vi "GetLocalizedPhraseLowLevel.vi"(7 "Dictionary":T1, 8 "error in (no error)":errorcluster, 10 "Target Language":string, 11 "Key":string) -> (0 "error out":errorcluster, 3 "Localized Phrase":string)   [LabVIEW 2017, in "JKI Simple Localization.lvlib"]
uses:
  API/JKI Simple Localization.lvlib
  Definitions/Dictionary--Cluster.ctl
  Definitions/Private/Font -- Cluster.ctl
  Definitions/Private/Phrase Dictionary Entry -- Cluster.ctl
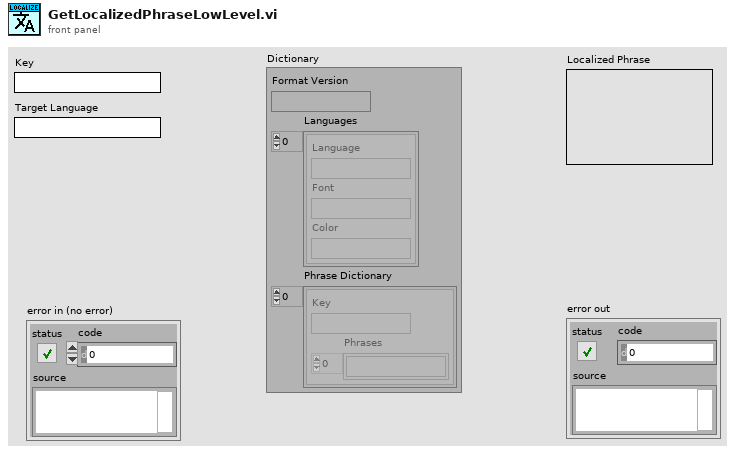
[diagram p1: front panel]
types:
  T1 = typedef "JKI Simple Localization.lvlib/Dictionary--Cluster.ctl" = cluster{"Format Version":string, "Languages":T2[], "Phrase Dictionary":T3[]}
  T2 = typedef "JKI Simple Localization.lvlib/Font -- Cluster.ctl" = cluster{"Language":string, "Font":string, "Color":string}
  T3 = typedef "JKI Simple Localization.lvlib/Phrase Dictionary Entry -- Cluster.ctl" = cluster{"Key":string, "Phrases":string[]}
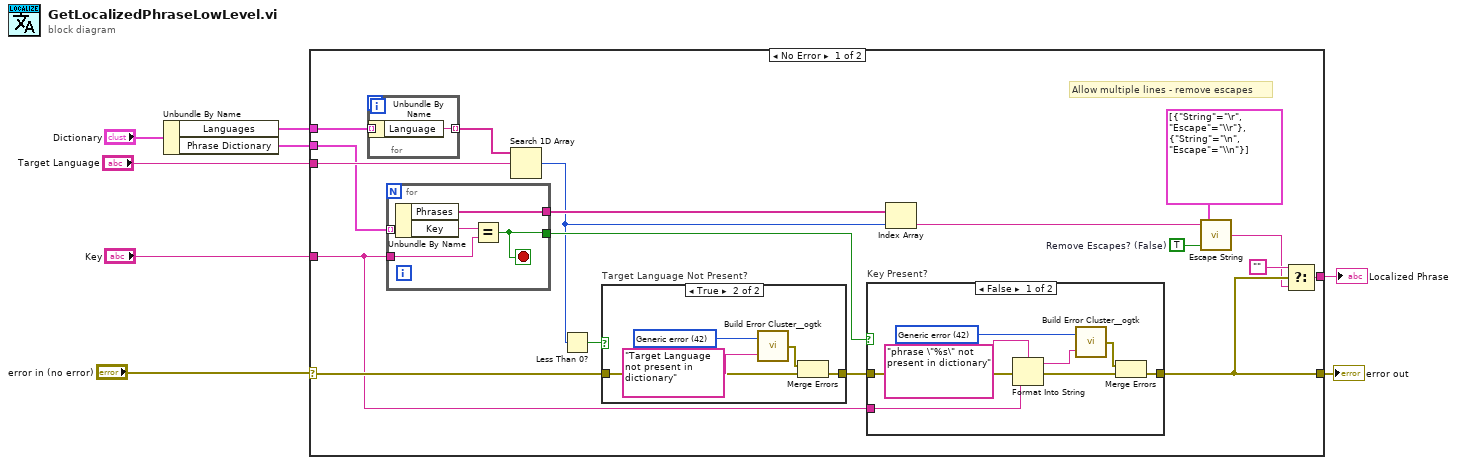
[diagram p0: block diagram]
diagram:
  n1 = Unbundle By Name("Dictionary") -> ("Languages"=w3:T2[], "Phrase Dictionary"=w1:T3[])
  n2 = case shown="No Error" "error in (no error)" {
    selector: "error in (no error)" -> [w22 w49]
    tunnel: w3 -> [w10 _]
    tunnel: [w12 _] -> w8
    tunnel: [w15 w49] -> w7
    tunnel: "Target Language" -> [w21 _]
    tunnel: "Key" -> [w11 _]
    tunnel: w1 -> [w16 _]
    frame No Error {
      w24 = TRUE  # Remove Escapes? (False)
      # "Allow multiple lines - remove escapes"
      n3 = for {
        tunnel: w10 -> [w28] mode=indexing
        tunnel: [w27] -> w9 mode=indexing
        n4 = Unbundle By Name(w28) -> ("Language"=w27:string)
      }
      n5 = for {
        tunnel: w16 -> [w33] mode=indexing
        tunnel: w11 -> [w31]
        tunnel: [w30] -> w19
        tunnel: [w29] -> w20
        stop <- w30 stop-if-true
        n6 = Unbundle By Name(w33) -> ("Phrases"=w29:string[], "Key"=w32:string)
        n7 = Equal?(x=w32, y=w31) -> (x = y?=w30:bool)
      }
      n8 = Search 1D Array(1D array=w9, element=w21) -> (index of element=w18:i32)  [unwired: 1 in]
      n9 = Less Than 0?(x=w18) -> (x < 0?=w26:bool)
      n10 = case "Target Language Not Present?" shown="True" w26 {
        tunnel: w22 -> [w43 w45]
        tunnel: [w43 w44] -> w25
        frame False {
        }
        frame True {
          w48 = 42 items=["No error", "Argument error", "Memory is full", "Out of zone", "End of file", "File already open", "Generic file I/O error", "File not found", "File permission error", "Disk is full", "Duplicate path", "Too many files open", "System feature not enabled", "Resource file not found", "Cannot add resource", "Resource not found", "Image not found", "Image memory error", "Pen does not exist", "Config type invalid", "Config token not found", "Config parse error", "Config memory error", "Bad external code format", "Bad external code offset", "External code not present", "Null window", "Destroy window error", "Null menu", "Print aborted", "Bad print record", "Print driver error", "Windows error during printing", "Memory error during printing", "Print dialog error", "Generic print error", "Invalid device refnum", "Device not found", "Device parameter error", "Device unit error", "Cannot open device", "Device call aborted", "Generic error", "Cancelled by user", "Object ID too low", "Object ID too high", "Object not in heap", "Unknown heap", "Unknown object (invalid DefProc)", "Unknown object (DefProc not in table)", "Message out of range", "Invalid (null) method", "Unknown message", "Manager call not supported", "Bad address", "Network operation in progress", "Network operation timed out", "Connection is busy", "Network attribute not supported", "Network error", "Address in use", "System out of memory", "Connection aborted", "Connection refused", "Not connected", "Already connected", "Connection closed", "Initialization error (interapplication manager)", "Bad occurrence", "Wait on unbound occurrence handler", "Occurrence queue overflow", "Datalog type conflict", "Unused", "Unrecognized type (interapplication manager)", "Memory corrupt", "Failed to make temporary DLL", "Old CIN version", "Drag socket not found", "Failed to load drop-object", "Failed to register OLE object", "Failed to release OLE object", "Format specifier type mismatch", "Unknown format specifier", "Too few format specifiers", "Too many format specifiers", "Scan failed", "Newer CIN version", "Error converting to variant", "Runtime menu error", "Password tampered", "Variant attribute not found", "Incompatible variant data type", "Event data is not available", "Event Store is not present", "Occurrence is not found", "Event Queue is not created", "Event info is not available", "Refnum passed is NULL", "Error retrieving Class GUID", "Error retrieving CoClass GUID", "Error retrieving TypeLib GUID.", "Bad built application magic bytes.", "Specific driver is different from the specific driver associated with the Logical Name.", "There is no session opened to the class driver.", "Max Error", "MAX - Error with config objects", "MAX - Error loading configuration", "MAX - Group not supported"]
          n11 = call <userlib>:"Build Error Cluster__ogtk.vi"("String to Prepend to source (\"\")"="Target Language not present in dictionary" ("String to Prepend to source (\"\")"), "code"=w48) -> ("error out"=w46:errorcluster)
          n12 = Merge Errors(w46, w45) -> (w44:errorcluster)
        }
      }
      n13 = case "Key Present?" shown="False" w19 {
        tunnel: w25 -> [w38 w42]
        tunnel: [w39 w42] -> w15
        tunnel: w11 -> [w35 _]
        frame False {
          w41 = 42 items=["No error", "Argument error", "Memory is full", "Out of zone", "End of file", "File already open", "Generic file I/O error", "File not found", "File permission error", "Disk is full", "Duplicate path", "Too many files open", "System feature not enabled", "Resource file not found", "Cannot add resource", "Resource not found", "Image not found", "Image memory error", "Pen does not exist", "Config type invalid", "Config token not found", "Config parse error", "Config memory error", "Bad external code format", "Bad external code offset", "External code not present", "Null window", "Destroy window error", "Null menu", "Print aborted", "Bad print record", "Print driver error", "Windows error during printing", "Memory error during printing", "Print dialog error", "Generic print error", "Invalid device refnum", "Device not found", "Device parameter error", "Device unit error", "Cannot open device", "Device call aborted", "Generic error", "Cancelled by user", "Object ID too low", "Object ID too high", "Object not in heap", "Unknown heap", "Unknown object (invalid DefProc)", "Unknown object (DefProc not in table)", "Message out of range", "Invalid (null) method", "Unknown message", "Manager call not supported", "Bad address", "Network operation in progress", "Network operation timed out", "Connection is busy", "Network attribute not supported", "Network error", "Address in use", "System out of memory", "Connection aborted", "Connection refused", "Not connected", "Already connected", "Connection closed", "Initialization error (interapplication manager)", "Bad occurrence", "Wait on unbound occurrence handler", "Occurrence queue overflow", "Datalog type conflict", "Unused", "Unrecognized type (interapplication manager)", "Memory corrupt", "Failed to make temporary DLL", "Old CIN version", "Drag socket not found", "Failed to load drop-object", "Failed to register OLE object", "Failed to release OLE object", "Format specifier type mismatch", "Unknown format specifier", "Too few format specifiers", "Too many format specifiers", "Scan failed", "Newer CIN version", "Error converting to variant", "Runtime menu error", "Password tampered", "Variant attribute not found", "Incompatible variant data type", "Event data is not available", "Event Store is not present", "Occurrence is not found", "Event Queue is not created", "Event info is not available", "Refnum passed is NULL", "Error retrieving Class GUID", "Error retrieving CoClass GUID", "Error retrieving TypeLib GUID.", "Bad built application magic bytes.", "Specific driver is different from the specific driver associated with the Logical Name.", "There is no session opened to the class driver.", "Max Error", "MAX - Error with config objects", "MAX - Error loading configuration", "MAX - Group not supported"]
          n14 = Format Into String(format string="phrase \"%s\" not present in dictionary" ("String to Prepend to source (\"\")"), error in=w38, w35) -> (resulting string=w34:string, error out=w37:errorcluster)  [unwired: 1 in]
          n15 = call <userlib>:"Build Error Cluster__ogtk.vi"("String to Prepend to source (\"\")"=w34, "code"=w41) -> ("error out"=w40:errorcluster)
          n16 = Merge Errors(w40, w37) -> (w39:errorcluster)
        }
        frame True {
        }
      }
      n17 = Index Array(array=w20, index=w18) -> (element=w17:string)
      n18 = call <vilib>:"Escape String.vi"("Remove Escapes? (False)"=w24, "Escapes"=cluster{"String":string, "Escape":string}[] [{"String"="\r", "Escape"="\\r"}, {"String"="\n", "Escape"="\\n"}], "String in"=w17) -> ("String out"=w13:string)
      n19 = Select(t="", s=w15, f=w13) -> (s? t:f=w12:string)
    }
    frame Error {
    }
  }
  "Localized Phrase" <- w8
  "error out" <- w7
